vi "GT_SetStopDec.vi"(8 "decSmoothStop":dbl, 9 "decAbruptStop":dbl, 10 "Profile in":i16, 11 "rtn_In":cluster{"rtn":i16, "Func":string}) -> (2 "Profile out":i16, 3 "rtn_Out":cluster{"rtn":i16, "Func":string})   [LabVIEW 2014]
uses:
  VC6/gts.dll
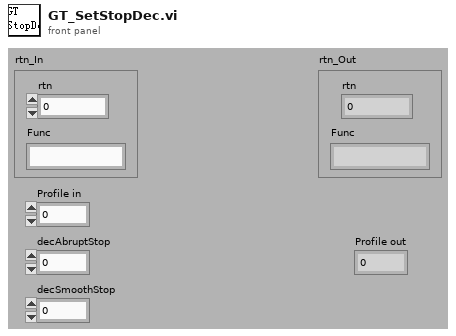
[diagram p1: front panel]
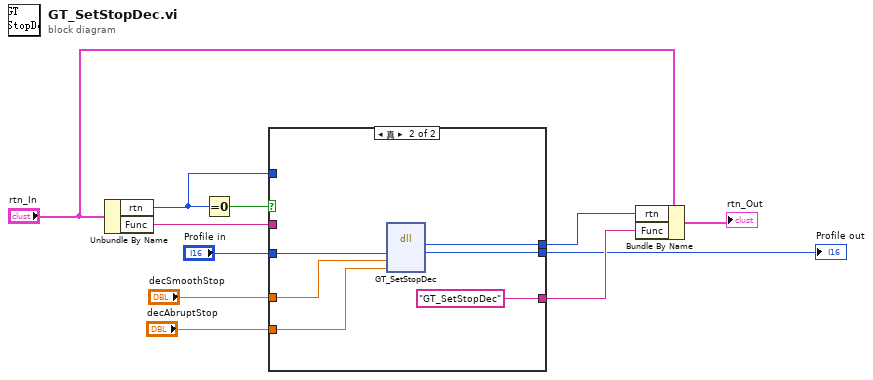
[diagram p0: block diagram]
diagram:
  n1 = Unbundle By Name("rtn_In") -> ("rtn"=w9:i16, "Func"=w10:string)
  n2 = Equal To 0?(x=w9) -> (x = 0?=w11:bool)
  n3 = case shown="真" w11 {
    tunnel: w10 -> [w13 _]
    tunnel: w9 -> [w14 _]
    tunnel: "Profile in" -> [w12 w20]
    tunnel: "decSmoothStop" -> [_ w19]
    tunnel: "decAbruptStop" -> [_ w18]
    tunnel: [w14 w17] -> w3
    tunnel: [w13 "GT_SetStopDec" ("Func")] -> w2
    tunnel: [w12 w15] -> w1
    frame False {
    }
    frame True {
      n4 = dll-call lib="PTH2Fabs DNewGTS AC-800LWin7版源程序-20170926gts85VC6gts.dll" fn="GT_SetStopDec"("Profile"=w20, "decSmoothStop"=w19, "decAbruptStop"=w18) -> ("rtn"=w17:i16, "Profile"=w15:i16)  [unwired: 5 in, 2 out]
    }
  }
  "Profile out" <- w1
  n5 = Bundle By Name(cluster="rtn_In", "rtn"=w3, "Func"=w2) -> (→"rtn_Out":cluster{"rtn":i16, "Func":string})
